vi "FlatToRichnidaqmx_grpc_CreateCIFreqChanRequest.vi"(5 "OutputClusterType":T1, 11 "InputCluster":T3) -> (3 "OutputCluster":T1)   [LabVIEW 2021, in "NI_DAQmx_client.lvlib"]
uses:
  NI_DAQmx_client.lvlib
  nidaqmx_grpc_CreateCIFreqChanRequest_units_enum/nidaqmx_grpc_CreateCIFreqChanRequest_units_enum.lvclass
  nidaqmx_grpc_CreateCIFreqChanRequest_edge_enum/nidaqmx_grpc_CreateCIFreqChanRequest_edge_enum.lvclass
  nidaqmx_grpc_CreateCIFreqChanRequest_meas_method_enum/nidaqmx_grpc_CreateCIFreqChanRequest_meas_method_enum.lvclass
  nidevice_grpc_Session_session/nidevice_grpc_Session_session.lvclass
  nidevice_grpc_Session.ctl
  nidaqmx_grpc_CreateCIFreqChanRequest.ctl
  nidaqmx_grpc_CounterFrequencyMethod.ctl
  nidaqmx_grpc_Edge1.ctl
  nidaqmx_grpc_FrequencyUnits3.ctl
  nidevice_grpc_Session_Flat.ctl
  nidaqmx_grpc_CreateCIFreqChanRequest_Flat.ctl
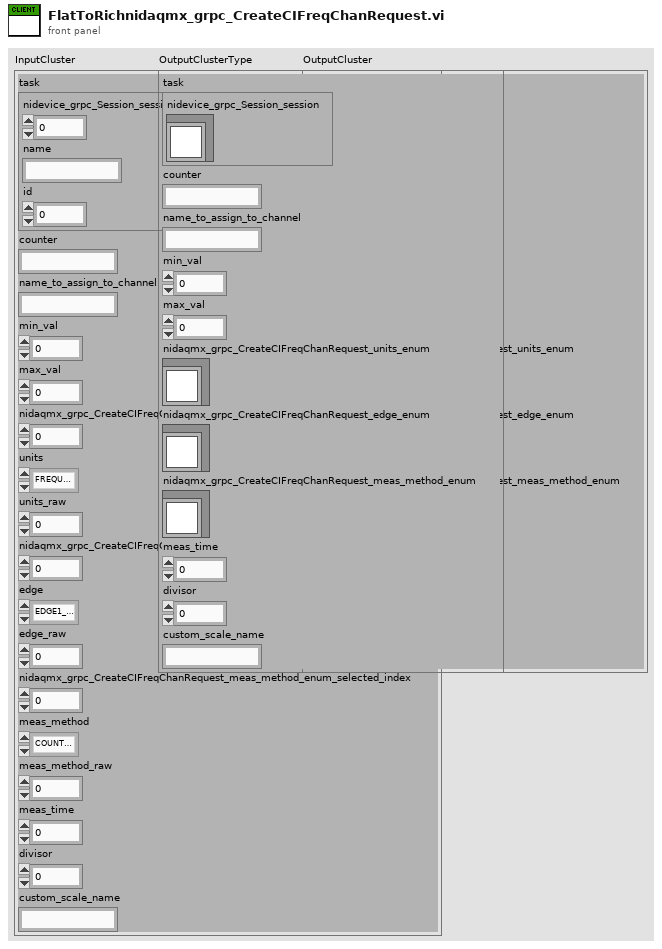
[diagram p1: front panel]
types:
  T1 = typedef "NI_DAQmx_client.lvlib/nidaqmx_grpc_CreateCIFreqChanRequest.ctl" = cluster{"task":T2, "counter":string, "name_to_assign_to_channel":string, "min_val":dbl, "max_val":dbl, "nidaqmx_grpc_CreateCIFreqChanRequest_units_enum":refnum<class "nidaqmx_grpc_CreateCIFreqChanRequest_units_enum.lvclass">, "nidaqmx_grpc_CreateCIFreqChanRequest_edge_enum":refnum<class "nidaqmx_grpc_CreateCIFreqChanRequest_edge_enum.lvclass">, "nidaqmx_grpc_CreateCIFreqChanRequest_meas_method_enum":refnum<class "nidaqmx_grpc_CreateCIFreqChanRequest_meas_method_enum.lvclass">, "meas_time":dbl, "divisor":u32, "custom_scale_name":string}
  T2 = typedef "NI_DAQmx_client.lvlib/nidevice_grpc_Session.ctl" = cluster{"nidevice_grpc_Session_session":refnum<class "nidevice_grpc_Session_session.lvclass">}
  T3 = typedef "NI_DAQmx_client.lvlib/nidaqmx_grpc_CreateCIFreqChanRequest_Flat.ctl" = cluster{"task":T4, "counter":string, "name_to_assign_to_channel":string, "min_val":dbl, "max_val":dbl, "nidaqmx_grpc_CreateCIFreqChanRequest_units_enum_selected_index":i32, "units":T5, "units_raw":i32, "nidaqmx_grpc_CreateCIFreqChanRequest_edge_enum_selected_index":i32, "edge":T6, "edge_raw":i32, "nidaqmx_grpc_CreateCIFreqChanRequest_meas_method_enum_selected_index":i32, "meas_method":T7, "meas_method_raw":i32, "meas_time":dbl, "divisor":u32, "custom_scale_name":string}
  T4 = typedef "NI_DAQmx_client.lvlib/nidevice_grpc_Session_Flat.ctl" = cluster{"nidevice_grpc_Session_session_selected_index":i32, "name":string, "id":u32}
  T5 = typedef "NI_DAQmx_client.lvlib/nidaqmx_grpc_FrequencyUnits3.ctl" = enum32{"FREQUENCY_UNITS3_UNSPECIFIED", "FREQUENCY_UNITS3_HZ", "FREQUENCY_UNITS3_TICKS", "FREQUENCY_UNITS3_FROM_CUSTOM_SCALE"}
  T6 = typedef "NI_DAQmx_client.lvlib/nidaqmx_grpc_Edge1.ctl" = enum32{"EDGE1_UNSPECIFIED", "EDGE1_RISING", "EDGE1_FALLING"}
  T7 = typedef "NI_DAQmx_client.lvlib/nidaqmx_grpc_CounterFrequencyMethod.ctl" = enum32{"COUNTER_FREQUENCY_METHOD_UNSPECIFIED", "COUNTER_FREQUENCY_METHOD_LOW_FREQ_1_CTR", "COUNTER_FREQUENCY_METHOD_HIGH_FREQ_2_CTR", "COUNTER_FREQUENCY_METHOD_LARGE_RNG_2_CTR", "COUNTER_FREQUENCY_METHOD_DYN_AVG"}
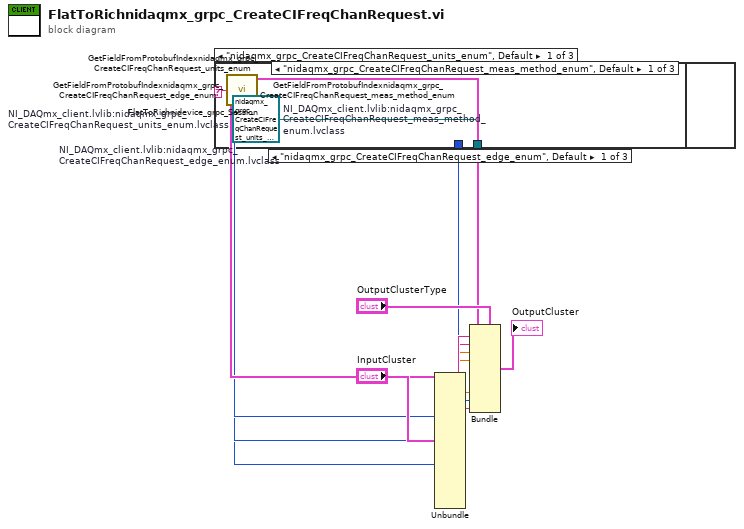
[diagram p0: block diagram]
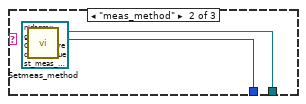
[diagram p2: hidden frame]
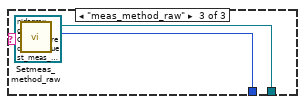
[diagram p3: hidden frame]
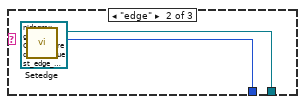
[diagram p4: hidden frame]
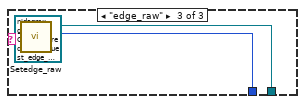
[diagram p5: hidden frame]
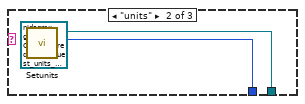
[diagram p6: hidden frame]
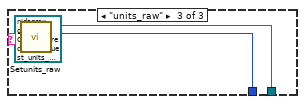
[diagram p7: hidden frame]
diagram:
  n1 = Unbundle "Unbundle"("InputCluster") -> ("task"=w24:T4, "counter"=w22:string, "name_to_assign_to_channel"=w21:string, "min_val"=w20:dbl, "max_val"=w19:dbl, "nidaqmx_grpc_CreateCIFreqChanRequest_units_enum_selected_index"=w18:i32, "units"=w15:T5, "units_raw"=w14:i32, "nidaqmx_grpc_CreateCIFreqChanRequest_edge_enum_selected_index"=w13:i32, "edge"=w10:T6, "edge_raw"=w9:i32, "nidaqmx_grpc_CreateCIFreqChanRequest_meas_method_enum_selected_index"=w8:i32, "meas_method"=w5:T7, "meas_method_raw"=w4:i32, "meas_time"=w3:dbl, "divisor"=w2:u32, "custom_scale_name"=w1:string)
  n2 = call "GetFieldFromProtobufIndexnidaqmx_grpc_CreateCIFreqChanRequest_meas_method_enum.vi"("protobuf index"=w8) -> ("oneof field name"=w7:string)
  n3 = case "nidaqmx_grpc_CreateCIFreqChanRequest_meas_method_enum" shown="\"nidaqmx_grpc_CreateCIFreqChanRequest_meas_method_enum\", Default" w7 {
    tunnel: [w28 w30 w33] -> w6
    tunnel: w5 -> [_ w31 _]
    tunnel: w4 -> [_ _ w34]
    frame "nidaqmx_grpc_CreateCIFreqChanRequest_meas_method_enum", Default {
      w28 = refnum<class "nidaqmx_grpc_CreateCIFreqChanRequest_meas_method_enum.lvclass"> refnum  # NI_DAQmx_client.lvlib:nidaqmx_grpc_CreateCIFreqChanRequest_meas_method_enum.lvclass
    }
    frame "meas_method" {
      n4 = call "Setmeas_method.vi"("Set_Val"=w31, "OneOfTemplate in"=refnum<class "nidaqmx_grpc_CreateCIFreqChanRequest_meas_method_enum.lvclass"> refnum) -> ("OneOfTemplate out"=w30:refnum<class "nidaqmx_grpc_CreateCIFreqChanRequest_meas_method_enum.lvclass">)  [unwired: 8 in, 1 out]
    }
    frame "meas_method_raw" {
      n5 = call "Setmeas_method_raw.vi"("Set_Val"=w34, "OneOfTemplate in"=refnum<class "nidaqmx_grpc_CreateCIFreqChanRequest_meas_method_enum.lvclass"> refnum) -> ("OneOfTemplate out"=w33:refnum<class "nidaqmx_grpc_CreateCIFreqChanRequest_meas_method_enum.lvclass">)  [unwired: 8 in, 1 out]
    }
  }
  n6 = call "GetFieldFromProtobufIndexnidaqmx_grpc_CreateCIFreqChanRequest_edge_enum.vi"("protobuf index"=w13) -> ("oneof field name"=w12:string)
  n7 = case "nidaqmx_grpc_CreateCIFreqChanRequest_edge_enum" shown="\"nidaqmx_grpc_CreateCIFreqChanRequest_edge_enum\", Default" w12 {
    tunnel: [w35 w37 w40] -> w11
    tunnel: w10 -> [_ w38 _]
    tunnel: w9 -> [_ _ w41]
    frame "nidaqmx_grpc_CreateCIFreqChanRequest_edge_enum", Default {
      w35 = refnum<class "nidaqmx_grpc_CreateCIFreqChanRequest_edge_enum.lvclass"> refnum  # NI_DAQmx_client.lvlib:nidaqmx_grpc_CreateCIFreqChanRequest_edge_enum.lvclass
    }
    frame "edge" {
      n8 = call "Setedge.vi"("Set_Val"=w38, "OneOfTemplate in"=refnum<class "nidaqmx_grpc_CreateCIFreqChanRequest_edge_enum.lvclass"> refnum) -> ("OneOfTemplate out"=w37:refnum<class "nidaqmx_grpc_CreateCIFreqChanRequest_edge_enum.lvclass">)  [unwired: 8 in, 1 out]
    }
    frame "edge_raw" {
      n9 = call "Setedge_raw.vi"("Set_Val"=w41, "OneOfTemplate in"=refnum<class "nidaqmx_grpc_CreateCIFreqChanRequest_edge_enum.lvclass"> refnum) -> ("OneOfTemplate out"=w40:refnum<class "nidaqmx_grpc_CreateCIFreqChanRequest_edge_enum.lvclass">)  [unwired: 8 in, 1 out]
    }
  }
  n10 = call "GetFieldFromProtobufIndexnidaqmx_grpc_CreateCIFreqChanRequest_units_enum.vi"("protobuf index"=w18) -> ("oneof field name"=w17:string)
  n11 = case "nidaqmx_grpc_CreateCIFreqChanRequest_units_enum" shown="\"nidaqmx_grpc_CreateCIFreqChanRequest_units_enum\", Default" w17 {
    tunnel: [w42 w44 w47] -> w16
    tunnel: w15 -> [_ w45 _]
    tunnel: w14 -> [_ _ w48]
    frame "nidaqmx_grpc_CreateCIFreqChanRequest_units_enum", Default {
      w42 = refnum<class "nidaqmx_grpc_CreateCIFreqChanRequest_units_enum.lvclass"> refnum  # NI_DAQmx_client.lvlib:nidaqmx_grpc_CreateCIFreqChanRequest_units_enum.lvclass
    }
    frame "units" {
      n12 = call "Setunits.vi"("Set_Val"=w45, "OneOfTemplate in"=refnum<class "nidaqmx_grpc_CreateCIFreqChanRequest_units_enum.lvclass"> refnum) -> ("OneOfTemplate out"=w44:refnum<class "nidaqmx_grpc_CreateCIFreqChanRequest_units_enum.lvclass">)  [unwired: 8 in, 1 out]
    }
    frame "units_raw" {
      n13 = call "Setunits_raw.vi"("Set_Val"=w48, "OneOfTemplate in"=refnum<class "nidaqmx_grpc_CreateCIFreqChanRequest_units_enum.lvclass"> refnum) -> ("OneOfTemplate out"=w47:refnum<class "nidaqmx_grpc_CreateCIFreqChanRequest_units_enum.lvclass">)  [unwired: 8 in, 1 out]
    }
  }
  n14 = call "FlatToRichnidevice_grpc_Session.vi"("InputCluster"=w24) -> ("OutputCluster"=w23:T2)  [unwired: 10 in]
  n15 = Bundle "Bundle"(cluster="OutputClusterType", "task"=w23, "counter"=w22, "name_to_assign_to_channel"=w21, "min_val"=w20, "max_val"=w19, "nidaqmx_grpc_CreateCIFreqChanRequest_units_enum"=w16, "nidaqmx_grpc_CreateCIFreqChanRequest_edge_enum"=w11, "nidaqmx_grpc_CreateCIFreqChanRequest_meas_method_enum"=w6, "meas_time"=w3, "divisor"=w2, "custom_scale_name"=w1) -> (→"OutputCluster":T1)
